vi "pp3_log_fromStringArray_trial.vi"(9 "Input string array":string[](array[string])) -> (2 "Was TRIAL?":bool, 3 "Trial in":T1={"Trial Type Number"=1, "Trial Type"=enum."GO", "Trial Weight"=100, "Shock (mA)"=0.3, "Duration (ms)"=0.25, "Sound Type"=enum."04 FM Sweep", "Stim P1"=4000.0, "Stim P2"=0.0, "Stim P3"=0.0, "Stim P4"=2000.0, "DAQ Amplitude (V)"=0.25} {"DAQ Amplitude (V)" min=0.0 max=5.0 format="%_4g"; "Shock (mA)" min=-1.0 max=5.0; "Trial Weight" step=1; "Duration (ms)" min=0.0 max=1.0; "Trial Type Number" min=1 max=256 step=1})   [LabVIEW 2013]
uses:
  CTL_pp3g_Trial.ctl
  pp3_CTL_TrialType.ctl
  labolabo2/waveforms/WFTypes.ctl
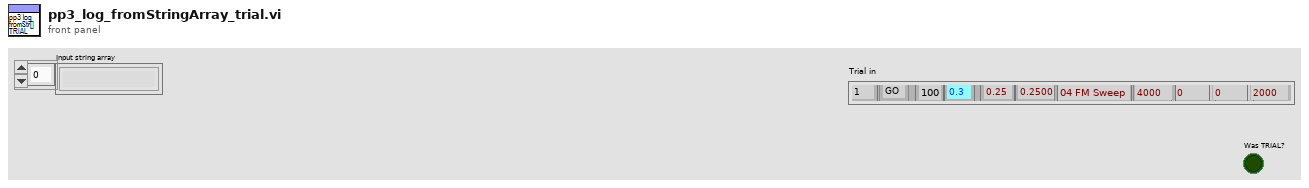
[diagram p1: front panel]
types:
  T1 = typedef "CTL_pp3g_Trial.ctl" = cluster{"Trial Type Number":i16, "Trial Type":T2, "Trial Weight":u32, "Shock (mA)":dbl, "Duration (ms)":dbl, "Sound Type":T3, "Stim P1":dbl, "Stim P2":dbl, "Stim P3":dbl, "Stim P4":dbl, "DAQ Amplitude (V)":dbl}
  T2 = typedef "pp3_CTL_TrialType.ctl" = enum16{"OFF", "GO", "NOGO", "TEST"}
  T3 = typedef "WFTypes.ctl" = enum16{"00 NULL", "01 DC", "02 Noise", "03 Pure Tone", "04 FM Sweep", "05 FM Sweep BURST"}
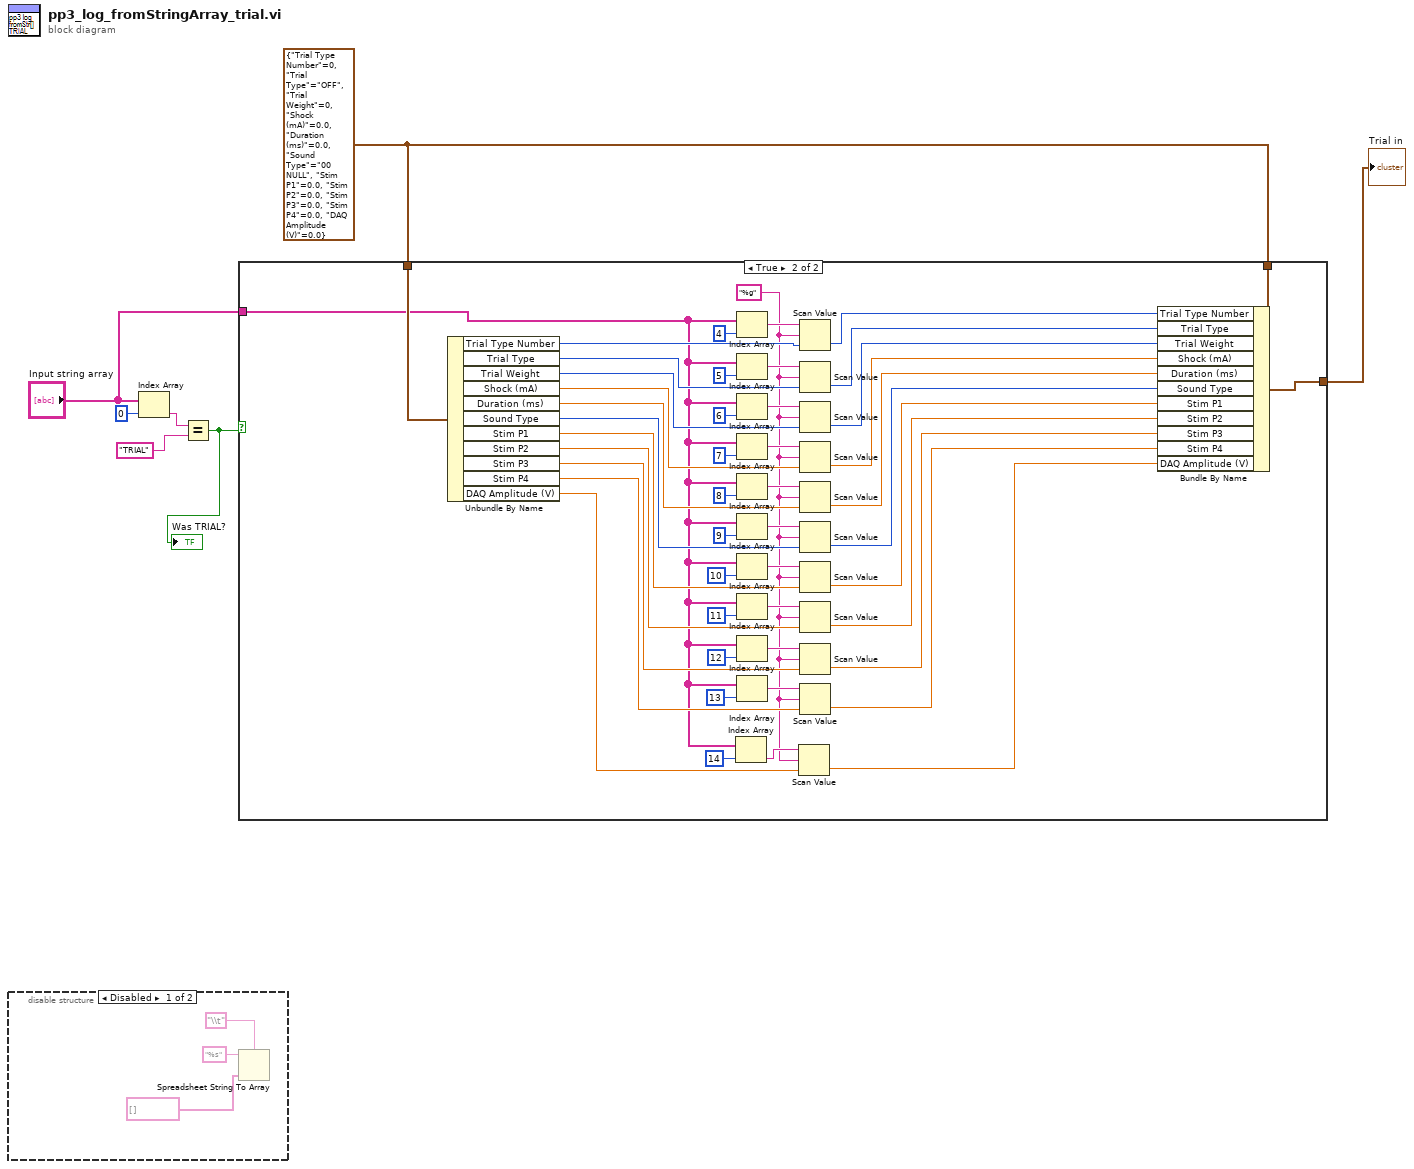
[diagram p0: block diagram]
diagram:
  w2 = T1 {"Trial Type Number"=0, "Trial Type"=enum."OFF", "Trial Weight"=0, "Shock (mA)"=0.0, "Duration (ms)"=0.0, "Sound Type"=enum."00 NULL", "Stim P1"=0.0, "Stim P2"=0.0, "Stim P3"=0.0, "Stim P4"=0.0, "DAQ Amplitude (V)"=0.0} ("Trial in")
  n1 = disable-structure shown="Disabled" {
    frame Disabled {
      n2 = Spreadsheet String To Array(delimiter (Tab)="\\t", format string="%s", array type (2D Dbl)=string[] [] ("appended array")) -> (spreadsheet string=w11:string)  [unwired: 1 out]
    }
    frame Enabled {
    }
  }
  n3 = Index Array(array="Input string array", index=0) -> (element=w5:string)
  n4 = Equal?(x=w5, y="TRIAL" ("element")) -> (x = y?=w1:bool)
  "Was TRIAL?" <- w1
  n5 = case shown="True" w1 {
    tunnel: w2 -> [w12 w61]
    tunnel: [w12 w60] -> w7
    tunnel: "Input string array" -> [_ w14]
    tunnel: w2 -> [_ w57]
    frame False {
    }
    frame True {
      w16 = "%g" ("format string")
      n6 = Unbundle By Name(w57) -> ("Trial Type Number"=w55:i16, "Trial Type"=w50:T2, "Trial Weight"=w49:u32, "Shock (mA)"=w40:dbl, "Duration (ms)"=w39:dbl, "Sound Type"=w38:T3, "Stim P1"=w30:dbl, "Stim P2"=w29:dbl, "Stim P3"=w28:dbl, "Stim P4"=w27:dbl, "DAQ Amplitude (V)"=w13:dbl)
      n7 = Index Array(array=w14, index=14) -> (element=w17:string)
      n8 = Index Array(array=w14, index=4) -> (element=w58:string)
      n9 = Index Array(array=w14, index=5) -> (element=w53:string)
      n10 = Index Array(array=w14, index=6) -> (element=w51:string)
      n11 = Index Array(array=w14, index=7) -> (element=w45:string)
      n12 = Index Array(array=w14, index=8) -> (element=w43:string)
      n13 = Index Array(array=w14, index=9) -> (element=w41:string)
      n14 = Index Array(array=w14, index=10) -> (element=w19:string)
      n15 = Index Array(array=w14, index=11) -> (element=w35:string)
      n16 = Index Array(array=w14, index=12) -> (element=w33:string)
      n17 = Index Array(array=w14, index=13) -> (element=w31:string)
      n18 = Scan Value(string=w17, format string=w16, default (0 dbl)=w13) -> (value=w15:dbl)  [unwired: 1 out]
      n19 = Scan Value(string=w58, format string=w16, default (0 dbl)=w55) -> (value=w56:i16)  [unwired: 1 out]
      n20 = Scan Value(string=w53, format string=w16, default (0 dbl)=w50) -> (value=w48:T2)  [unwired: 1 out]
      n21 = Scan Value(string=w51, format string=w16, default (0 dbl)=w49) -> (value=w47:u32)  [unwired: 1 out]
      n22 = Scan Value(string=w45, format string=w16, default (0 dbl)=w40) -> (value=w26:dbl)  [unwired: 1 out]
      n23 = Scan Value(string=w43, format string=w16, default (0 dbl)=w39) -> (value=w25:dbl)  [unwired: 1 out]
      n24 = Scan Value(string=w41, format string=w16, default (0 dbl)=w38) -> (value=w24:T3)  [unwired: 1 out]
      n25 = Scan Value(string=w19, format string=w16, default (0 dbl)=w30) -> (value=w23:dbl)  [unwired: 1 out]
      n26 = Scan Value(string=w35, format string=w16, default (0 dbl)=w29) -> (value=w22:dbl)  [unwired: 1 out]
      n27 = Scan Value(string=w33, format string=w16, default (0 dbl)=w28) -> (value=w21:dbl)  [unwired: 1 out]
      n28 = Scan Value(string=w31, format string=w16, default (0 dbl)=w27) -> (value=w20:dbl)  [unwired: 1 out]
      n29 = Bundle By Name(cluster=w61, "Trial Type Number"=w56, "Trial Type"=w48, "Trial Weight"=w47, "Shock (mA)"=w26, "Duration (ms)"=w25, "Sound Type"=w24, "Stim P1"=w23, "Stim P2"=w22, "Stim P3"=w21, "Stim P4"=w20, "DAQ Amplitude (V)"=w15) -> (w60:T1)
    }
  }
  "Trial in" <- w7
